vi "AlliGator Clear Variables.vi"(8 "Error In":errorcluster) -> (0 "Error Out":errorcluster, 1 "Message":string)   [LabVIEW 2021, in "AlliGator Globals, Variables & Constants.lvlib"]
doc: "Reset all internal variables to their default."
uses:
  AlliGator Globals, Variables & Constants.lvlib
  AlliGator Variables List.ctl
  Python Plugins API/AlliGator Python Plugins.lvlib
  Error/Error.lvlib
panel:
  in  "Alligator Variable":T1=enum."Phasor Plot:Image Reference Points"
  # "see the AlliGator License on the block diagram (Ctrl+E or Window:Show Block Diagram)"
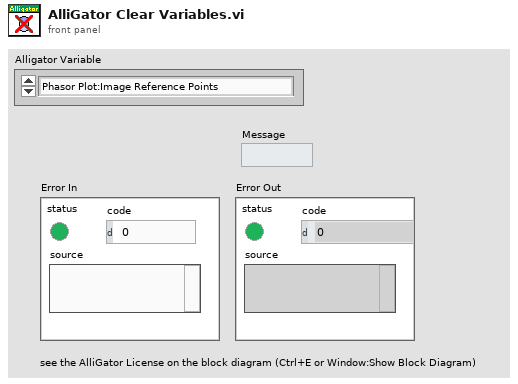
[diagram p1: front panel]
types:
  T1 = typedef "AlliGator Globals, Variables & Constants.lvlib/AlliGator Variables List.ctl" = enum16{"---- GUI ----", "GUI:Initialization Status", "GUI:State Indicators Refnum", "GUI:Original AlliGator Menu Items", "GUI:Current Action Loop State", "GUI:Script in progress", "GUI:Playback", "GUI:Loop Playback", "GUI:Search ROI Used", "GUI:Search ROI", "Decay Graph Max Legend Size", "Intensity Graph Max Legend Size", "Decay Statistics Graph Max Legend Size", "Phasor Graph Max Legend Size", "Phasor Ratio Graph Max Legend Size", "Lifetime Graph Max Legend Size", "---- Files ----", "Files:Export Dataset Frames as Individual Files", "Files:Show Batch Export Help Balloons", "Files:Frames in Dataset", "Files:ptu File Frame Start Indices", "Files:Current Frame in Dataset", "Files:Current Frame Timestamp", "Files:Dataset Loaded", "Files:Dataset Metadata", "Files:Dataset Channel", "Files:Dataset Data Description", "Files:Background Dataset Metadata", "Files:Background Dataset Channel", "Files:Background Dataset Data Description", "Files:Background File Subtraction", "Files:Background File Path", "Files:Background File Pile-up Correction", "Files:Background File Pixel Well Capacity", "Files:Background File Scaling Factor", "Files:Current Dataset Load Settings", "Files:Dataset Path", "Files:ICCD-specific Information", "Files:Macrotime Gate Separation", "------ Python Plugins ------", "Python Plugins:Information", "Python Plugins:Python Session", "Python Plugins:Valid Python Session?", "---- Source Image ----", "Source Image:ROIs", "Source Image:Current ROI", "Source Image:ROI Event Refnum", "X_Source Image Display Range", "X_Source Image Palette Information", "X_Type of Displayed Image", "X_Time Gate Slider", "Source Image:Palette List", "Source Image:Scale", "Source Image:ROI Overlay Color", "Source Image:Overlay to Erase", "Source Image:Is Displayed Image Accumulated", "Source Image:White Light Image Modified", "Source Image:Mask Image Modified", "---- Image Profile Window ----", "Image Profile:Window Event Refnum", "Image Profile:IntensityType", "Image Profile:Intensity Average Type", "Image Profile:Intensity-weighted SDV", "Image Profile:Box Profile Type", "Image Profile:Window Open", "Image Profile:Plotted Fit Parameter", "------ Phasor Graph -------", "Phasor Graph:Show Line", "---- Phasor Plot ---", "Phasor Plot:Parameters Changed", "Phasor Plot:FLI Dataset Modified since last Calculation", "Phasor Harmonics Data", "Selected Phasor Harmonics", "Phasor Harmonic Manager Event Refnum", "Phasor Plot:ROIs", "Phasor Plot:Current ROI", "Phasor Plot:ROI Event Refnum", "Phasor Plot:Image Reference Points", "Phasor Plot:Computed", "Phasor Plot:Palette Information", "Phasor Plot:Palette List", "Phasor Plot:Phasor Ratio Palette Information", "Phasor Plot:Phasor Ratio Palette List", "Phasor Plot:Image Scale", "Phasor Plot:Image Overlay to Erase", "Phasor Plot:Image Elements to Update", "Phasor Plot:Current Calculation Parameters", "Phasor Plot:Current Calibration Options", "Phasor Plot:Reset Cumulated Phasor Plot", "Phasor Plot:Reference 1", "Phasor Plot:Lifetime Reference 1", "Phasor Plot:Reference 1 Frequency", "Phasor Plot:Reference 2", "Phasor Plot:Lifetime Reference 2", "Phasor Plot:Reference 2 Frequency", "---- Decay Analysis ----", "Number of Selected Decays to Fit", "LS Fit Results", "LAR Fit Results", "BS Fit Results", "Last Decay Max - Min", "Best Fit Parameters", "Best Fit Parameter Names", "Actual Size X", "Actual Size Y", "Binning X", "Binning Y", "Actual # Gates", "Dataset Number", "Gates to...", "Gates Skipped", "Gates to keep", "Gate Step", "Gate Separation", "Reversed Gates", "Pile-up Correction", "Pixel Well Capacity", "Background Subtracted", "Background Subtraction Method", "Background Definition Range", "Background File (deprecated)", "Number of Dataset Accumulated", "Array of Accumulated Dataset Paths", "Do Averaged Datasets", "Destination File Path", "Process Plot Target", "Use 1/D as Phasor Frequency", "---- Decay Fit Parameter Map -----", "Decay Fit Parameter Map:Palette Information", "Decay Fit Parameter Map:Palette List", "---- Parameter Map ----", "Parameter Map:Palette Information", "Parameter Map:Palette List", "------- Local Decay Window ---------", "Local Decay Graph Window:Event Refnum", "Local Decay Graph Window:Use normalized IRF for convolution", "----- Miscellaneous ----", "Misc:Skippable Dialog Windows Status"}
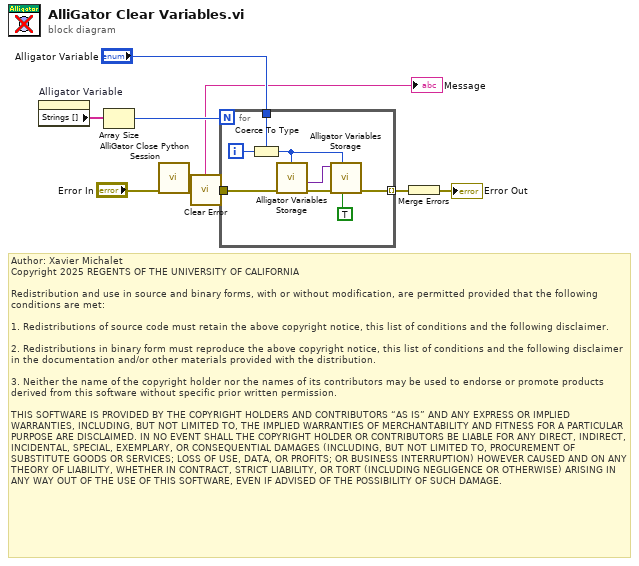
[diagram p0: block diagram]
diagram:
  # "Author: Xavier Michalet\nCopyright 2025 REGENTS OF THE UNIVERSITY OF CALIFORNIA\n\nRedistribution and use in source and binary forms, with or without modification, are permitted provided that the following conditions are met:\n\n1. Redistributions of source code must retain the above copyright notice, this list of conditions and the following disclaimer.\n\n2. Redistributions in binary form must reproduce the above copyright notice, this list of conditions and the following disclaimer in the documentation and/or other materials provided with the distribution.\n\n3. Neither the name of the copyright holder nor the names of its contributors may be used to endorse or promote products derived from this software without specific prior written permission.\n\nTHIS SOFTWARE IS PROVIDED BY THE COPYRIGHT HOLDERS AND CONTRIBUTORS “AS IS” AND ANY EXPRESS OR IMPLIED WARRANTIES, INCLUDING, BUT NOT LIMITED TO, THE IMPLIED WARRANTIES OF MERCHANTABILITY AND FITNESS FOR A PARTICULAR PURPOSE ARE DISCLAIMED. IN NO EVENT SHALL THE COPYRIGHT HOLDER OR CONTRIBUTORS BE LIABLE FOR ANY DIRECT, INDIRECT, INCIDENTAL, SPECIAL, EXEMPLARY, OR CONSEQUENTIAL DAMAGES (INCLUDING, BUT NOT LIMITED TO, PROCUREMENT OF SUBSTITUTE GOODS OR SERVICES; LOSS OF USE, DATA, OR PROFITS; OR BUSINESS INTERRUPTION) HOWEVER CAUSED AND ON ANY THEORY OF LIABILITY, WHETHER IN CONTRACT, STRICT LIABILITY, OR TORT (INCLUDING NEGLIGENCE OR OTHERWISE) ARISING IN ANY WAY OUT OF THE USE OF THIS SOFTWARE, EVEN IF ADVISED OF THE POSSIBILITY OF SUCH DAMAGE."
  n1 = property on="Alligator Variable" class="Enum (strict)"() -> ("Strings []"=w9:string[])  [unwired: 2 in, 2 out]
  n2 = Array Size(array=w9) -> (size(s)=w8:i32)
  n3 = call "AlliGator Close Python Session.vi"("Error In"="Error In") -> ("Error Out"=w3:errorcluster, "Message"=→"Message":string)  [unwired: 9 in]
  n4 = call "Clear Error.vi"("Error In"=w3) -> ("no Error Out"=w2:errorcluster)  [unwired: 8 in]
  n5 = for {
    N: w8 -> [_]
    tunnel: [w16] -> w7 mode=indexing
    tunnel: w2 -> [w11]
    tunnel: "Alligator Variable" -> [w15]
    i -> [w17]
    n6 = Coerce To Type(0:w17, 1:w15) -> (2:w14:T1)
    n7 = call "Alligator Variables Storage.vi"("AlliGator Variable"=w14, "Error In"=w11) -> ("Error Out"=w12:errorcluster, "Default Data out"=w13:variant)  [unwired: 7 in, 1 out]
    n8 = call "Alligator Variables Storage.vi"("Get(F)/Set"=TRUE, "AlliGator Variable"=w14, "Error In"=w12, "Data in"=w13) -> ("Error Out"=w16:errorcluster)  [unwired: 5 in, 2 out]
  }
  n9 = Merge Errors(w7) -> (→"Error Out":errorcluster)
